vi "Day 12.vi"() -> ()   [LabVIEW 2023]
panel:
  in  "input":string="abccccaaacaccccaaaaacccccccaaccccccccaaaaaaccccccaaaaaccccccccccaaaaaaaaacccccccaaaaaaaaaaaaaaccaaaaaccccccccccccaccacccccccccccccccccccccccccccccccccccccccaaaaaa\nabccaacaaaaaccaaaaacccccaaaaaccccccccaaaaaaccccccaaaaaacccccccccaaaaaaaaaaaaacccaaaaaaaaaaaaaaaaaaaaaccccccccccccaaaacccccccccccccccccccccccccccccccccccccccaaaaaa\nabccaaaaaaaaccaaaaaacccccaaaaaccccccaaaaaaaacccccaaaaaaccccccccccaaaaaaaaaaaacccaaaaaacaaaaaacaaaaaaaaccccccccccaaaaacccccaccccccccccccccccccaaacccccccccccccaaaaa\nabcccaaaaaccccccaaaacccccaaaaacccccaaaaaaaaaaccccaaaaaacccccccccaaaaaaaaaaaaaacaaaaaaaaaaaaaacaaaaaaaaccccccccc..."
  out "Visited":bool[][](array[boolean])
  out "Distance":u32
  out "E+Z":T1
  out "Intensity Graph":i32[][](graph)
  in  "test":bool
  in  "test input":string="Sabqponm\nabcryxxl\naccszExk\nacctuvwj\nabdefghi\n"
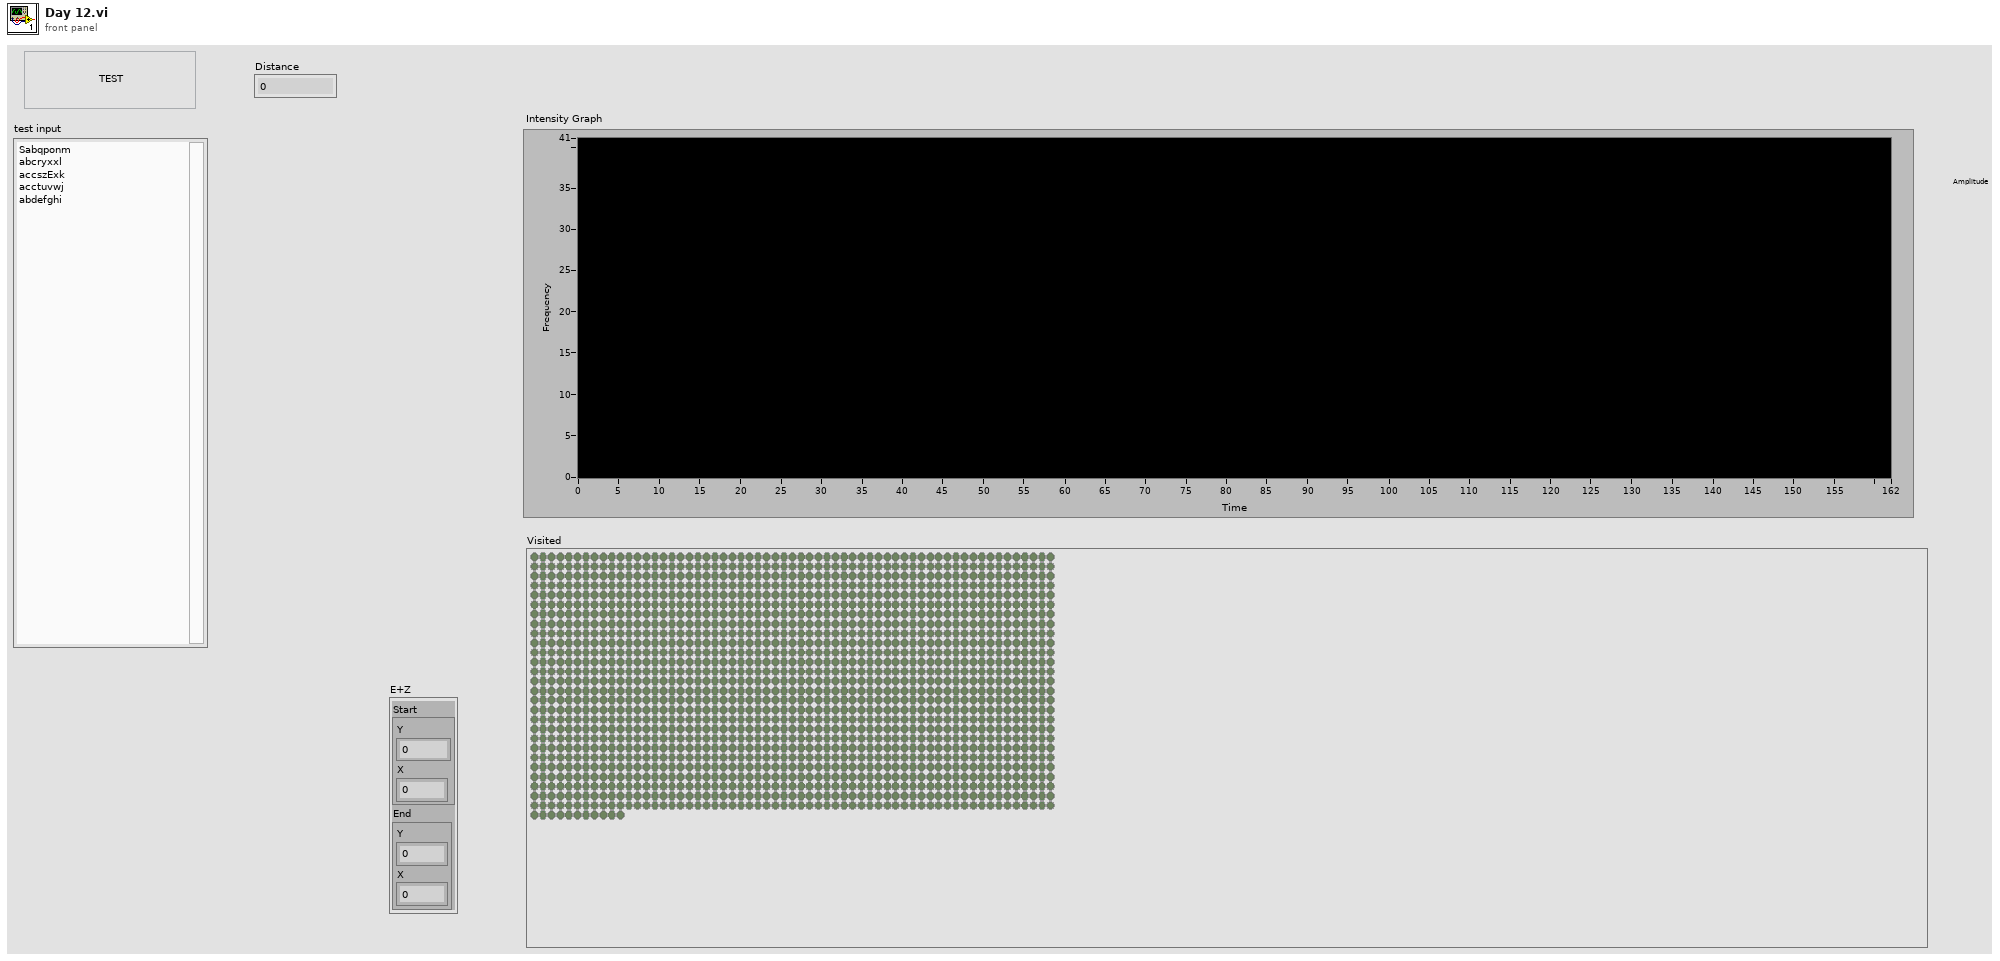
[diagram p1: front panel]
types:
  T1 = cluster{"Start":cluster{"Y":i32, "X":i32}, "End":cluster{"Y":i32, "X":i32}}
  T2 = cluster{"Distance":u32, "point":cluster{"Y":i32, "X":i32}}
  T3 = cluster{"Distance":u32, "point":cluster{"Y":i32, "X":i32}, "previus point":cluster{"Y":i32, "X":i32}, "Level":i32, "visited":bool}
  T4 = cluster{"Distance":u32, "point":cluster{"Y":i32, "X":i32}, "previus point":cluster{"Y":i32, "X":i32}, "Level":i32, "visited":bool}[][]
  T5 = cluster{"Distance":u32, "point":cluster{"Y":i32, "X":i32}}[]
  T6 = cluster{"Distance":u32, "Priority\nQueue":cluster{"Distance":u32, "point":cluster{"Y":i32, "X":i32}}}
  T7 = cluster{"Distance":u32, "Priority\nQueue":cluster{"Distance":u32, "point":cluster{"Y":i32, "X":i32}}}[]
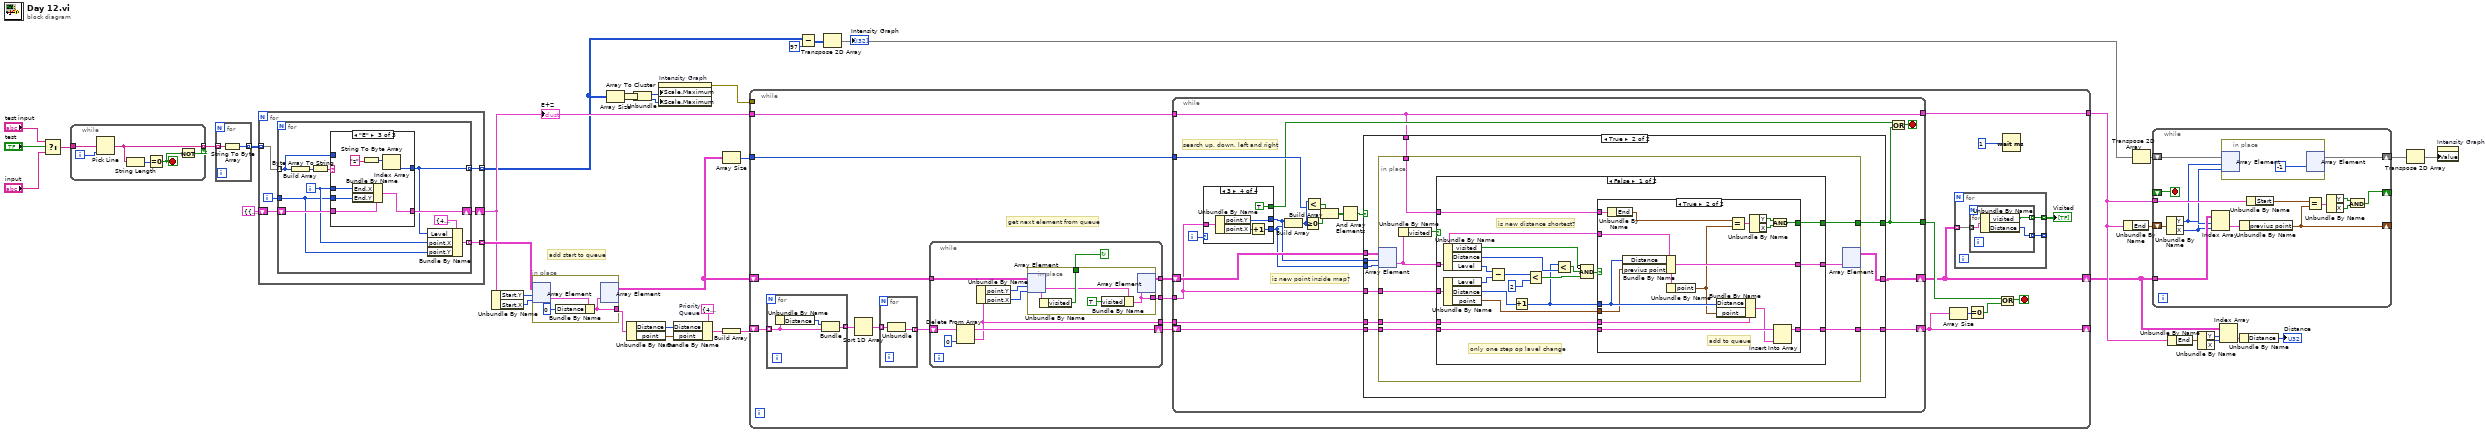
[diagram p0: block diagram]
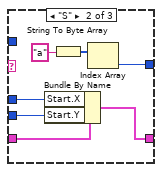
[diagram p3: hidden frame]
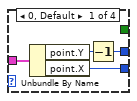
[diagram p7: hidden frame]
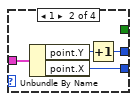
[diagram p8: hidden frame]
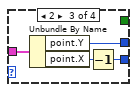
[diagram p9: hidden frame]
diagram:
  w27 = T2 {"Distance"=4294967295, "point"={"Y"=0, "X"=0}}  # Priority Queue
  # "add start to queue"
  n1 = Select(t="test input", s="test", f="input") -> (s? t:f=w38:string)
  n2 = while {
    tunnel: w38 -> [w43]
    tunnel: [w42] -> w35 mode=indexing if=w40
    i -> [w44]
    stop <- w41 stop-if-true
    n3 = Pick Line(multi-line string=w43, line index=w44) -> (output string=w42:string)  [unwired: 1 in]
    n4 = String Length(string=w42) -> (length=w45:i32)
    n5 = Equal To 0?(x=w45) -> (x = 0?=w41:bool)
    n6 = Not(x=w41) -> (.not. x?=w40:bool)
  }
  n7 = for {
    tunnel: w35 -> [w47] mode=indexing
    tunnel: [w46] -> w32 mode=indexing
    n8 = String To Byte Array(string=w47) -> (unsigned byte array=w46:u8[])
  }
  n9 = for {
    tunnel: w32 -> [w53] mode=indexing
    shift-right: [w50] -> w15
    shift-left: T1 {"Start"={"Y"=0, "X"=0}, "End"={"Y"=0, "X"=0}} -> [w52]
    tunnel: [w49] -> w6 mode=indexing
    tunnel: [w48] -> w29 mode=indexing
    i -> [w51]
    n10 = for {
      tunnel: w53 -> [w59] mode=indexing
      shift-right: [w60] -> w50
      shift-left: w52 -> [w61]
      tunnel: w51 -> [w55]
      tunnel: [w58] -> w49 mode=indexing
      tunnel: [w57] -> w48 mode=indexing
      i -> [w56]
      n11 = Build Array(w59) -> (w63:u8[])
      n12 = Byte Array To String(unsigned byte array=w63) -> (string=w62:string)
      n13 = case shown="\"E\"" w62 {
        tunnel: w61 -> [w65 w72 w79]
        tunnel: [w65 w71 w78] -> w60
        tunnel: w55 -> [_ w69 w77]
        tunnel: w56 -> [_ w70 w76]
        tunnel: [w64 w66 w73] -> w58
        tunnel: w59 -> [w64 _ _]
        frame "False", Default {
        }
        frame "S" {
          n14 = Bundle By Name(cluster=w72, "Start.X"=w70, "Start.Y"=w69) -> (w71:T1)
          n15 = String To Byte Array(string="a") -> (unsigned byte array=w67:u8[])
          n16 = Index Array(array=w67) -> (element=w66:u8)  [unwired: 1 in]
        }
        frame "E" {
          n17 = Bundle By Name(cluster=w79, "End.X"=w76, "End.Y"=w77) -> (w78:T1)
          n18 = String To Byte Array(string="z") -> (unsigned byte array=w74:u8[])
          n19 = Index Array(array=w74) -> (element=w73:u8)  [unwired: 1 in]
        }
      }
      n20 = Bundle By Name(cluster=T3 {"Distance"=4294967295, "point"={"Y"=0, "X"=0}, "previus point"={"Y"=-1, "X"=-1}, "Level"=0, "visited"=FALSE}, "Level"=w58, "point.X"=w56, "point.Y"=w55) -> (w57:T3)
    }
  }
  "E+Z" <- w15
  n21 = Unbundle By Name(w15) -> ("Start.Y"=w30:i32, "Start.X"=w28:i32)
  n22 = in-place {
    in-place-border: [w80] -> w26
    n23 = in-place-array #1(w29, w30, w28) -> (w82:T3)
    n24 = Bundle By Name(cluster=w82, "Distance"=u32 0) -> (w80:T3)
    n25 = in-place-array #1(w80) -> (w21:T4)  [unwired: 2 out]
  }
  n26 = Array Size(array=w6) -> (size(s)=w5:i32[])
  n27 = Array To Cluster(array=w5) -> (cluster=w4:cluster{"[0]":i32, "[1]":i32})
  n28 = Unbundle By Name(w26) -> ("Distance"=w24:u32, "point"=w25:cluster{"Y":i32, "X":i32})
  n29 = Unbundle(w4) -> ("[0]"=w3:i32, "[1]"=w2:i32)
  n30 = property on="Intensity Graph" class="IntGraph (strict)"("YScale.Maximum"=w3, "XScale.Maximum"=w2) -> (error out=w1:errorcluster)  [unwired: 2 in, 1 out]
  n31 = Bundle By Name(cluster=w27, "Distance"=w24, "point"=w25) -> (w23:T2)
  n32 = Build Array(w23) -> (w22:T5)
  n33 = Array Size(array=w21) -> (size(s)=w20:i32[])
  n34 = while {
    shift-right: [w89] -> _
    shift-left: w22 -> [w102]
    shift-right: [w91] -> w11
    shift-left: w21 -> [w98]
    tunnel: w20 -> [w94]
    tunnel: w15 -> [w84]
    tunnel: [w83] -> w12
    tunnel: w1 -> [_]
    stop <- w87 stop-if-true
    # "get next element from queue"
    n35 = for {
      tunnel: w102 -> [w120] mode=indexing
      tunnel: [w119] -> w101 mode=indexing
      n36 = Unbundle By Name(w120) -> ("Distance"=w121:u32)
      n37 = Bundle("Distance"=w121, "Priority\nQueue"=w120) -> (w119:T6)  [unwired: 1 in]
    }
    n38 = Sort 1D Array(array=w101) -> (sorted array=w100:T7)
    n39 = for {
      tunnel: w100 -> [w118] mode=indexing
      tunnel: [w117] -> w99 mode=indexing
      n40 = Unbundle(w118) -> ("Priority\nQueue"=w117:T2)  [unwired: 1 out]
    }
    n41 = while {
      shift-right: [w112] -> w95
      shift-left: w99 -> [w104]
      tunnel: w98 -> [w110]
      tunnel: [w105] -> w96
      tunnel: [w109] -> w97
      tunnel: [w111] -> w93
      stop <- w106 continue-if-true
      n42 = Delete From Array(array=w104, index=0) -> (deleted portion=w111:T2, array with subset deleted=w112:T5)  [unwired: 1 in]
      n43 = Unbundle By Name(w111) -> ("point.Y"=w108:i32, "point.X"=w107:i32)
      n44 = in-place {
        in-place-border: [w116] -> w106
        in-place-border: [w113] -> w105
        n45 = in-place-array #2(w110, w108, w107) -> (w115:T3)
        n46 = Unbundle By Name(w115) -> ("visited"=w116:bool)
        n47 = Bundle By Name(cluster=w115, "visited"=TRUE) -> (w113:T3)
        n48 = in-place-array #2(w113) -> (w109:T4)  [unwired: 2 out]
      }
    }
    n49 = while {
      tunnel: w96 -> [w125]
      tunnel: w94 -> [w135]
      tunnel: w93 -> [w128]
      tunnel: [w122] -> w92
      shift-right: [w129] -> w89
      shift-left: w95 -> [w130]
      shift-right: [w127] -> w91
      shift-left: w97 -> [w133]
      tunnel: w84 -> [w124]
      tunnel: [w124] -> w83
      i -> [w140]
      stop <- w123 stop-if-true
      # "search up, down, left and right"
      # "is new point inside map?"
      n50 = case shown="3" w140 {
        tunnel: w125 -> [w204 w208 w212 w217]
        tunnel: [w201 w205 w210 w215] -> w132
        tunnel: [w202 w206 w209 w214] -> w131
        tunnel: [_ _ _ TRUE] -> w126
        frame 0, Default {
          n51 = Unbundle By Name(w204) -> ("point.Y"=w203:i32, "point.X"=w202:i32)
          n52 = Decrement(x=w203) -> (x-1=w201:i32)
        }
        frame 1 {
          n53 = Unbundle By Name(w208) -> ("point.Y"=w207:i32, "point.X"=w206:i32)
          n54 = Increment(x=w207) -> (x+1=w205:i32)
        }
        frame 2 {
          n55 = Unbundle By Name(w212) -> ("point.Y"=w210:i32, "point.X"=w211:i32)
          n56 = Decrement(x=w211) -> (x-1=w209:i32)
        }
        frame 3 {
          n57 = Unbundle By Name(w217) -> ("point.Y"=w215:i32, "point.X"=w216:i32)
          n58 = Increment(x=w216) -> (x+1=w214:i32)
        }
      }
      n59 = Build Array(w132, w131) -> (w139:i32[])
      n60 = Greater Or Equal To 0?(x=w139) -> (x >= 0?=w137:bool[])
      n61 = Less?(x=w139, y=w135) -> (x < y?=w138:bool[])
      n62 = Build Array(w138, w137) -> (w136:bool[][])
      n63 = And Array Elements(Boolean array=w136) -> (logical AND=w134:bool)
      n64 = case shown="True" w134 {
        tunnel: w133 -> [w141 w152]
        tunnel: w132 -> [_ w151]
        tunnel: w131 -> [_ w150]
        tunnel: w125 -> [_ w149]
        tunnel: w130 -> [w142 w148]
        tunnel: [w142 w147] -> w129
        tunnel: w128 -> [_ w146]
        tunnel: [w141 w145] -> w127
        tunnel: [_ w144] -> w122
        tunnel: w124 -> [_ w143]
        frame False {
        }
        frame True {
          n65 = in-place {
            in-place-border: w149 -> [w158]
            in-place-border: w148 -> [w160]
            in-place-border: [w159] -> w147
            in-place-border: w146 -> [w157]
            in-place-border: [w156] -> w144
            in-place-border: w143 -> [w153]
            n66 = in-place-array #3(w152, w151, w150) -> (w155:T3)
            n67 = Unbundle By Name(w155) -> ("visited"=w154:bool)
            n68 = case shown="False" w154 {
              tunnel: w155 -> [w179 w200]
              tunnel: [w176 w200] -> w161
              tunnel: w160 -> [w175 w199]
              tunnel: [w174 w199] -> w159
              tunnel: w158 -> [w173 _]
              tunnel: w157 -> [w172 _]
              tunnel: [w167 _] -> w156
              tunnel: w153 -> [w162 _]
              frame False {
                # "is new distance shortest?"
                # "only one step op lavel change"
                n69 = Unbundle By Name(w179) -> ("visited"=w166:bool, "Distance"=w169:u32, "Level"=w165:i32)
                n70 = Unbundle By Name(w173) -> ("Level"=w181:i32, "Distance"=w164:u32, "point"=w177:cluster{"Y":i32, "X":i32})
                n71 = Subtract(x=w165, y=w181) -> (x-y=w163:i32)
                n72 = Increment(x=w164) -> (x+1=w168:u32)
                n73 = Less?(x=w163, y=2) -> (x < y?=w178:bool)
                n74 = Less?(x=w168, y=w169) -> (x < y?=w170:bool)
                n75 = Compound Arithmetic op=AND(invert w166, w170, w178) -> (w171:bool)
                n76 = case shown="True" w171 {
                  tunnel: w179 -> [w183 w198]
                  tunnel: w168 -> [_ w197]
                  tunnel: w177 -> [_ w196]
                  tunnel: [w183 w192] -> w176
                  tunnel: w175 -> [w182 w195]
                  tunnel: [w182 w194] -> w174
                  tunnel: w172 -> [_ w193]
                  tunnel: [_ w186] -> w167
                  tunnel: w162 -> [_ w184]
                  frame False {
                  }
                  frame True {
                    # "add to queue"
                    n77 = Unbundle By Name(w184) -> ("End"=w185:cluster{"Y":i32, "X":i32})
                    n78 = Bundle By Name(cluster=w198, "Distance"=w197, "previus point"=w196) -> (w192:T3)
                    n79 = Unbundle By Name(w192) -> ("point"=w187:cluster{"Y":i32, "X":i32})
                    n80 = Bundle By Name(cluster=w193, "Distance"=w197, "point"=w187) -> (w191:T2)
                    n81 = Equal?(x=w185, y=w187) -> (x = y?=w190:cluster{"Y":bool, "X":bool})
                    n82 = Unbundle By Name(w190) -> ("Y"=w189:bool, "X"=w188:bool)
                    n83 = And(x=w189, y=w188) -> (x .and. y?=w186:bool)
                    n84 = Insert Into Array(array=w195, new element=w191) -> (w194:T5)  [unwired: 1 in]
                  }
                }
              }
              frame True {
              }
            }
            n85 = in-place-array #3(w161) -> (w145:T4)  [unwired: 2 out]
          }
        }
      }
      n86 = Or(x=w126, y=w122) -> (x .or. y?=w123:bool)
    }
    n87 = Array Size(array=w89) -> (size(s)=w88:i32)
    n88 = for {
      tunnel: w91 -> [w220] mode=indexing
      tunnel: [w219] -> w90 mode=indexing
      tunnel: [w218] -> _ mode=indexing
      n89 = for {
        tunnel: w220 -> [w223] mode=indexing
        tunnel: [w222] -> w219 mode=indexing
        tunnel: [w221] -> w218 mode=indexing
        n90 = Unbundle By Name(w223) -> ("visited"=w222:bool, "Distance"=w221:u32)
      }
    }
    "Visited" <- w90
    n91 = Equal To 0?(x=w88) -> (x = 0?=w86:bool)
    n92 = Or(x=w92, y=w86) -> (x .or. y?=w87:bool)
    n93 = Wait (ms)(milliseconds to wait=u32 1) -> ()  [unwired: 1 out]
  }
  n94 = Subtract(x=w6, y=97 ("Numeric")) -> (x-y=w31:i32[][])
  n95 = Transpose 2D Array(2D array=w31) -> (transposed array=w10:i32[][])
  "Intensity Graph" <- w10
  n96 = Unbundle By Name(w12) -> ("End"=w13:cluster{"Y":i32, "X":i32})
  n97 = Transpose 2D Array(2D array=w10) -> (transposed array=w8:i32[][])
  n98 = while {
    tunnel: w11 -> [w238]
    shift-right: [w230] -> _
    shift-left: w13 -> [w237]
    tunnel: w12 -> [w232]
    shift-right: [w228] -> w9
    shift-left: w8 -> [w229]
    shift-right: [w225] -> _
    shift-left: _ -> [w224]
    stop <- w224 stop-if-true
    n99 = Unbundle By Name(w237) -> ("Y"=w227:i32, "X"=w226:i32)
    n100 = Index Array(array=w238, index (row)=w227, index (col)=w226) -> (element=w236:T3)
    n101 = in-place {
      n102 = in-place-array #4(w229, w227, w226) -> ()  [unwired: 1 out]
      n103 = in-place-array #4(-1 ("x")) -> (w228:i32[][])  [unwired: 2 out]
    }
    n104 = Unbundle By Name(w236) -> ("previus point"=w230:cluster{"Y":i32, "X":i32})
    n105 = Unbundle By Name(w232) -> ("Start"=w231:cluster{"Y":i32, "X":i32})
    n106 = Equal?(x=w231, y=w230) -> (x = y?=w233:cluster{"Y":bool, "X":bool})
    n107 = Unbundle By Name(w233) -> ("Y"=w234:bool, "X"=w235:bool)
    n108 = And(x=w234, y=w235) -> (x .and. y?=w225:bool)
  }
  n109 = Unbundle By Name(w12) -> ("End"=w14:cluster{"Y":i32, "X":i32})
  n110 = Unbundle By Name(w14) -> ("Y"=w19:i32, "X"=w18:i32)
  n111 = Index Array(array=w11, index (row)=w19, index (col)=w18) -> (element=w17:T3)
  n112 = Unbundle By Name(w17) -> ("Distance"=→"Distance":u32)
  n113 = Transpose 2D Array(2D array=w9) -> (transposed array=w7:i32[][])
  n114 = property on="Intensity Graph" class="IntGraph (strict)"("Value"=w7) -> ()  [unwired: 2 in, 2 out]
